vi "Config Dialog.vi"(10 "Container State":T2 caption="container state", 11 "state in":T3={"Draw Options"={"Text Color"=16777238, "Wing Color"=16751616, "Dial Outline Color"=13816530, "Sky Color"=3381759, "Ground Color"=8213043, "Horizon Line Color"=16777225, "Outline Color"=0, "Dial Background Color"=5987163, "Draw Wings"=TRUE, "Draw Text"=TRUE, "Font Name"="Helvetica", "Angle units"=enum."Radians"}} caption="State") -> (0 "state changed?":bool, 1 "data changed?":bool, 3 "state out":T3={"Draw Options"={"Text Color"=16777238, "Wing Color"=16751616, "Dial Outline Color"=13816530, "Sky Color"=3381759, "Ground Color"=8213043, "Horizon Line Color"=16777225, "Outline Color"=0, "Dial Background Color"=5987163, "Draw Wings"=TRUE, "Draw Text"=TRUE, "Font Name"="Helvetica", "Angle units"=enum."Radians"}} caption="State")   [LabVIEW 2017, in "Attitude Indicator.xctl"]
uses:
  <vilib>/robotics/Controls/Attitude Indicator/Attitude Indicator.xctl
  <vilib>/robotics/Controls/Utilities/Color Box_No Transparent.ctl
  <vilib>/robotics/Controls/Utilities/Color Box.ctl
  <vilib>/robotics/Controls/Attitude Indicator/_Attitude Indicator Support Files/Attitude Indicator State.ctl
  <vilib>/robotics/Controls/Attitude Indicator/Attitude Picture/Draw Options.ctl
  <vilib>/robotics/Controls/Utilities/Angle Units.ctl
  <vilib>/_xctls/Container State.ctl
  <vilib>/robotics/Controls/Attitude Indicator/Attitude Picture/Attitude.ctl
  <vilib>/robotics/Controls/Attitude Indicator/Attitude Picture/NI_Robotics_Attitude Picture.lvlib
  <vilib>/_xctls/XControlSupport.lvlib
  <vilib>/robotics/Controls/Utilities/NI_Robotics_Control Utilities.lvlib
panel:
  in  "help":bool
  in  "cancel":bool
  in  "ok":bool
  in  "Angle Units":enum16{"Radians", "Degrees"}(ring)=enum."Degrees"
  in  "text":T1=16777238 caption="Text"
  out "2D Picture":picture
  in  "dial outline color":T1=13816530 caption="Dial Outline"
  in  "draw text":bool=TRUE caption="Draw Text"
  in  "draw wings":bool=TRUE caption="Draw Wings"
  in  "dial bkgnd color":T6=5987163 caption="Dial Background"
  in  "outline color":T6 caption="Outline"
  in  "horizon line color":T1=16777225 caption="Horizon Line"
  in  "ground color":T1=8213043 caption="Ground"
  in  "sky color":T1=3381759 caption="Sky"
  in  "wing color":T1=16751616 caption="Wings"
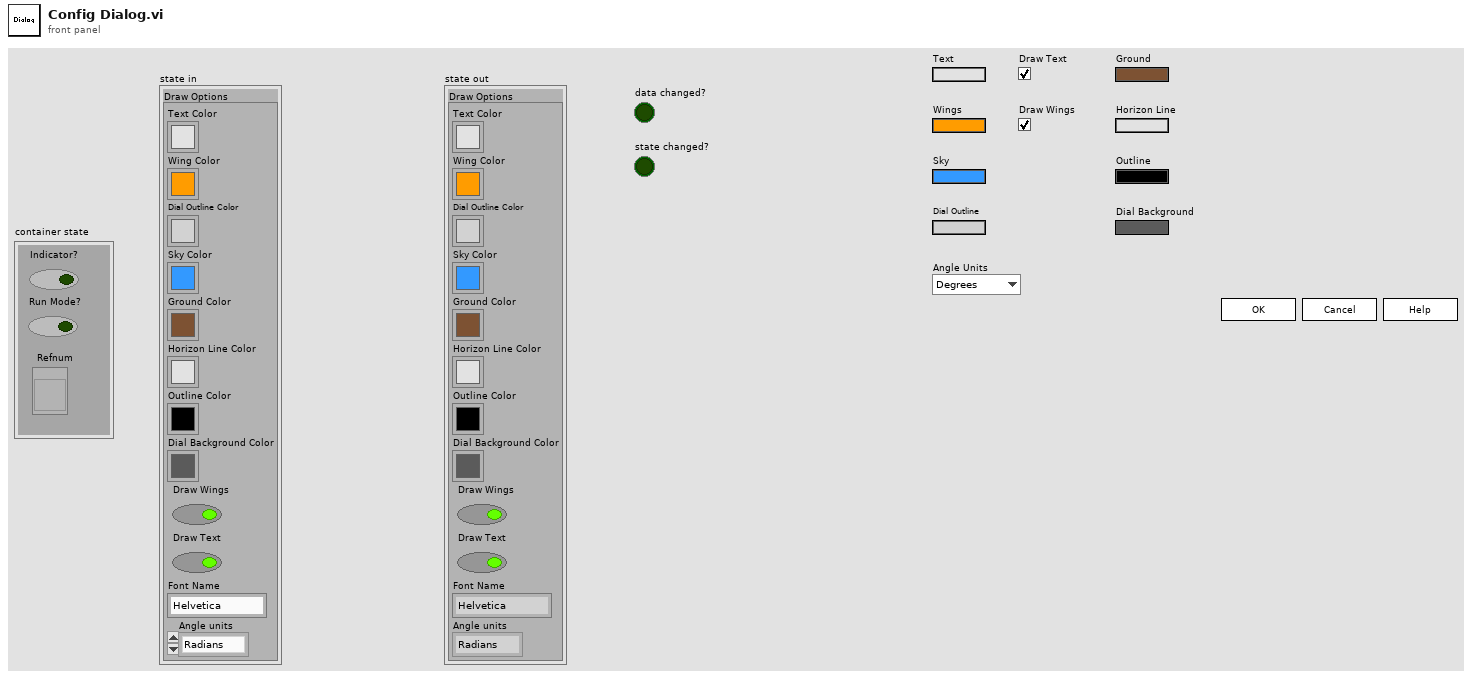
[diagram p1: front panel]
types:
  T1 = typedef "NI_Robotics_Control Utilities.lvlib/Color Box_No Transparent.ctl" = u32
  T2 = typedef "XControlSupport.lvlib/Container State.ctl" = cluster{"Indicator?":bool, "Run Mode?":bool, " Refnum":refnum<vi>}
  T3 = typedef "Attitude Indicator.xctl/Attitude Indicator State.ctl" = cluster{"Draw Options":T4}
  T4 = typedef "NI_Robotics_Attitude Picture.lvlib/Draw Options.ctl" = cluster{"Text Color":u32, "Wing Color":u32, "Dial Outline Color":u32, "Sky Color":u32, "Ground Color":u32, "Horizon Line Color":u32, "Outline Color":u32, "Dial Background Color":u32, "Draw Wings":bool, "Draw Text":bool, "Font Name":string, "Angle units":T5}
  T5 = typedef "NI_Robotics_Control Utilities.lvlib/Angle Units.ctl" = enum16{"Radians", "Degrees"}
  T6 = typedef "NI_Robotics_Control Utilities.lvlib/Color Box.ctl" = u32
  T7 = typedef "NI_Robotics_Attitude Picture.lvlib/Attitude.ctl" = cluster{"roll":dbl, "pitch":dbl}
  T8 = typedef "LVBoundsTypeDef.ctl" = cluster{"Width":u32, "Height":u32}
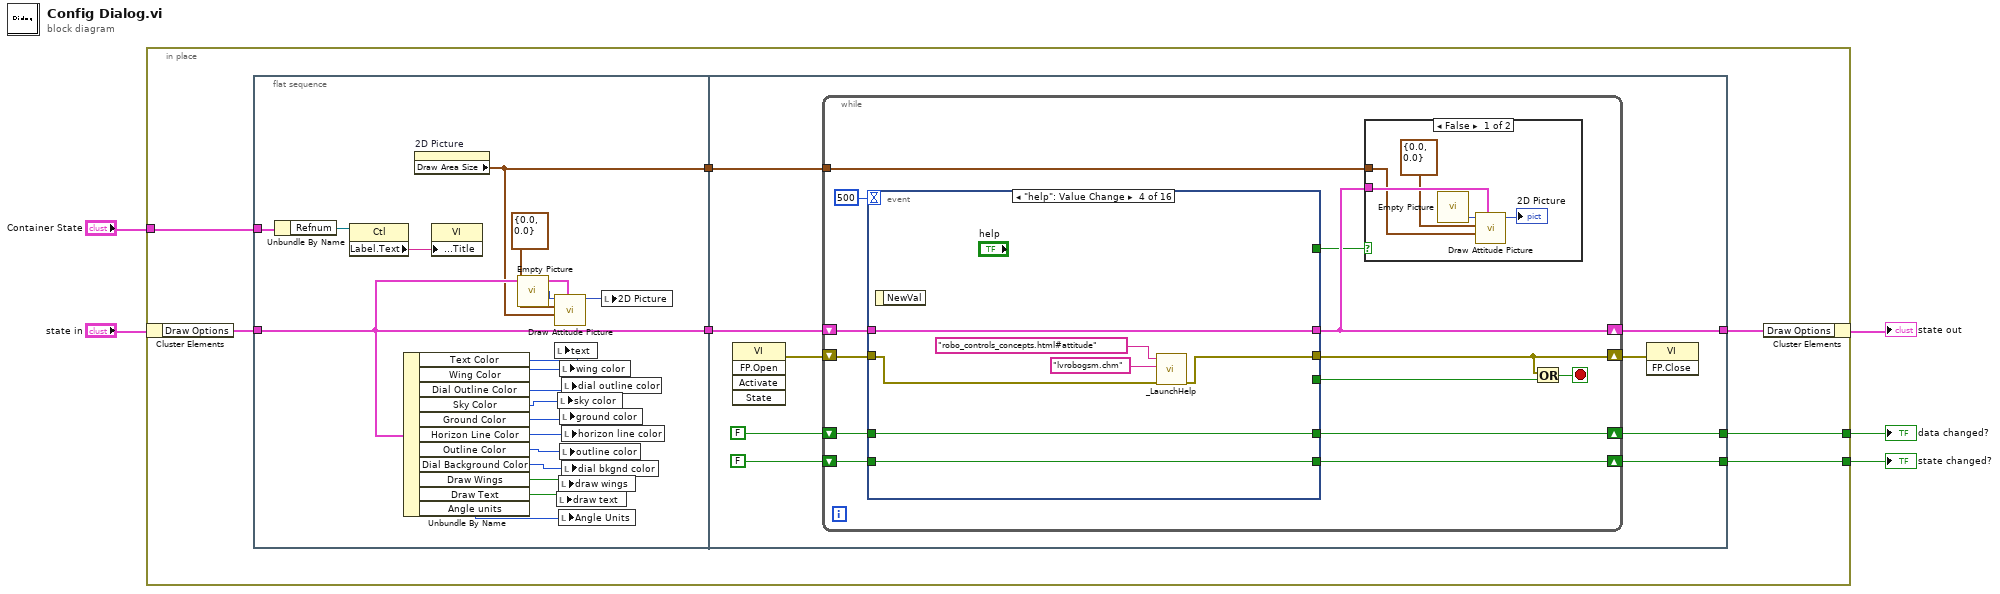
[diagram p0: block diagram]
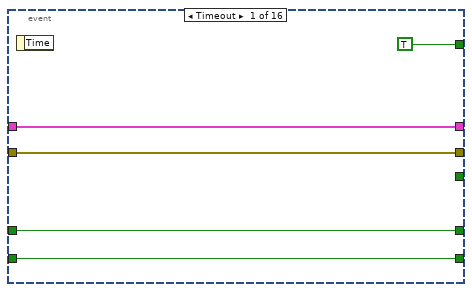
[diagram p3: hidden frame]
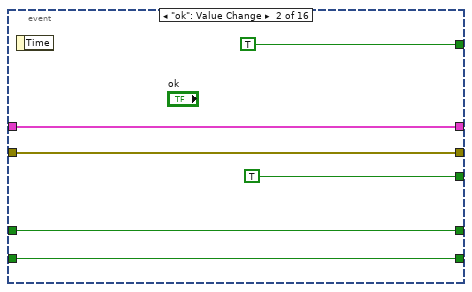
[diagram p4: hidden frame]
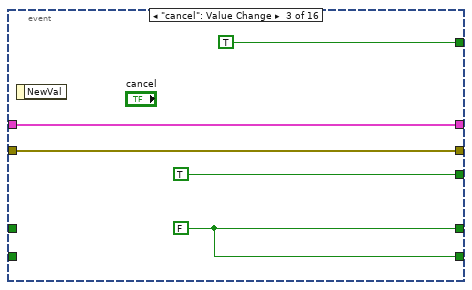
[diagram p5: hidden frame]
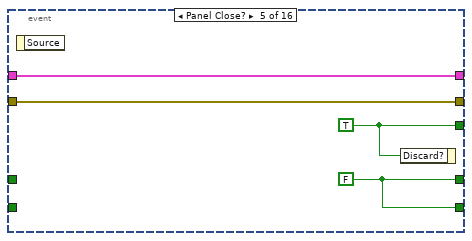
[diagram p6: hidden frame]
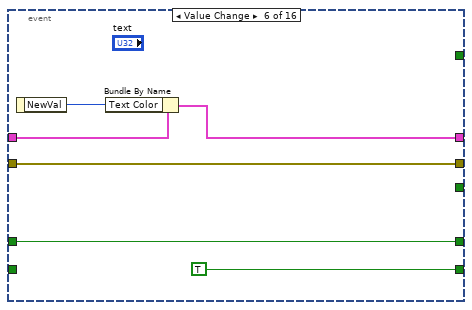
[diagram p7: hidden frame]
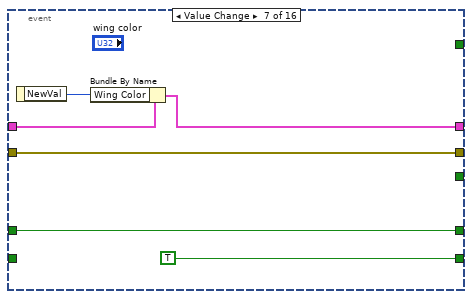
[diagram p8: hidden frame]
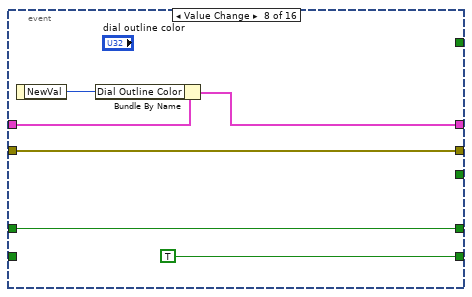
[diagram p9: hidden frame]
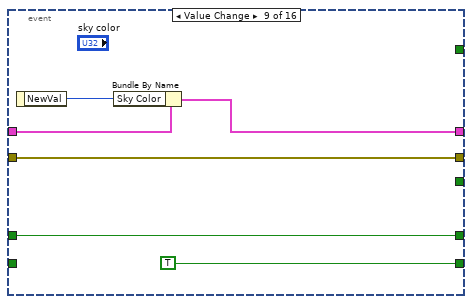
[diagram p10: hidden frame]
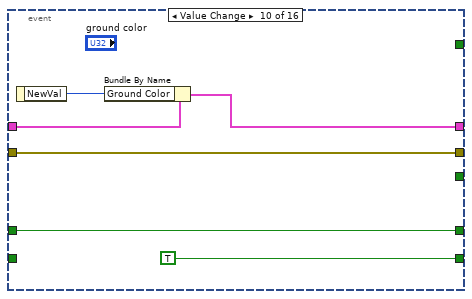
[diagram p11: hidden frame]
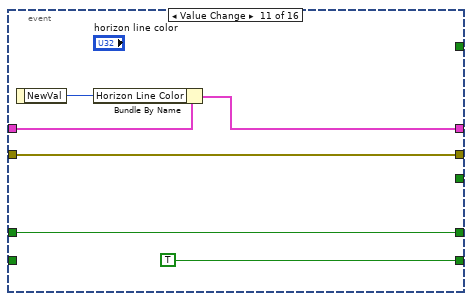
[diagram p12: hidden frame]
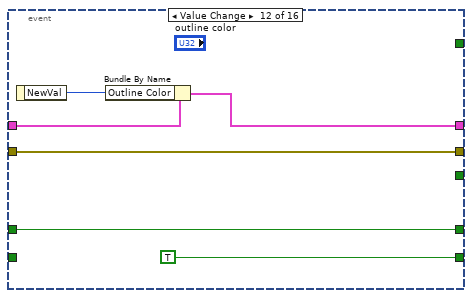
[diagram p13: hidden frame]
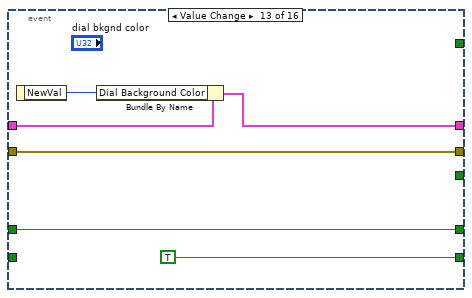
[diagram p14: hidden frame]
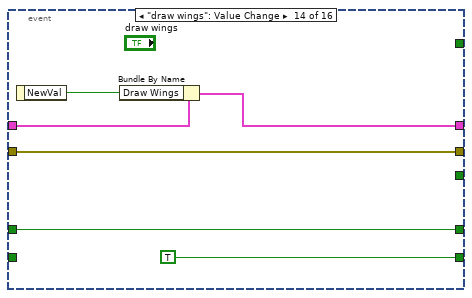
[diagram p15: hidden frame]
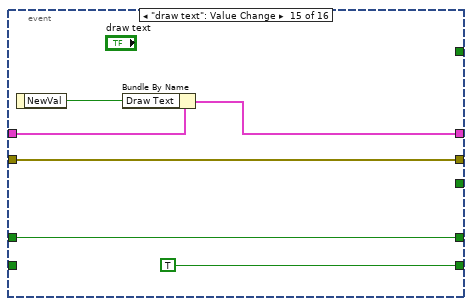
[diagram p16: hidden frame]
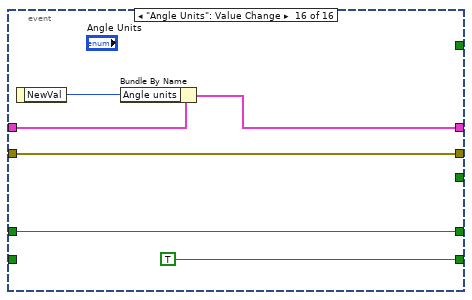
[diagram p17: hidden frame]
diagram:
  n1 = in-place {
    in-place-border: [w10] -> w5
    in-place-border: [w9] -> w4
    in-place-border: "Container State" -> [w6]
    n2 = in-place-cluster #1("state in") -> ("Draw Options"=w8:T4)
    n3 = flat-sequence {
      tunnel: w8 -> [w20]
      tunnel: [w20] -> w12
      tunnel: [w19] -> w11
      tunnel: w6 -> [w17]
      tunnel: [w39] -> w7
      tunnel: w12 -> [w40]
      tunnel: [w34] -> w10
      tunnel: [w33] -> w9
      tunnel: w11 -> [w32]
      frame #0 {
        n4 = Unbundle By Name(w17) -> ("Refnum"=w16:refnum<vi>)
        n5 = property class="Ctl"(reference=w16) -> ("Label.Text"=w15:string)  [unwired: 1 in, 2 out]
        n6 = Unbundle By Name(w20) -> ("Text Color"=w31:u32, "Wing Color"=w30:u32, "Dial Outline Color"=w29:u32, "Sky Color"=w28:u32, "Ground Color"=w27:u32, "Horizon Line Color"=w26:u32, "Outline Color"=w25:u32, "Dial Background Color"=w24:u32, "Draw Wings"=w23:bool, "Draw Text"=w22:bool, "Angle units"=w14:T5)
        n7 = property on="2D Picture" class="Pict"() -> ("Draw Area Size"=w19:T8)  [unwired: 2 in, 2 out]
        n8 = property class="VI"("Front Panel.Title"=w15) -> ()  [unwired: 2 in, 2 out]
        n9 = call "Empty Picture"() -> ("empty picture"=w18:picture)
        n10 = call <vilib>:"Draw Attitude Picture.vi"("draw options"=w20, "DrawAreaSize"=w19, "attitude"=T7 {"roll"=0.0, "pitch"=0.0}, "picture in"=w18) -> ("picture out"=w21:picture)  [unwired: 6 in, 1 out]
        n11 = local write "text"(w31) -> ()
        n12 = local write "draw text"(w22) -> ()
        n13 = local write "sky color"(w28) -> ()
        n14 = local write "draw wings"(w23) -> ()
        n15 = local write "Angle Units"(w14) -> ()
        n16 = local write "wing color"(w30) -> ()
        n17 = local write "ground color"(w27) -> ()
        n18 = local write "outline color"(w25) -> ()
        n19 = local write "dial outline color"(w29) -> ()
        n20 = local write "horizon line color"(w26) -> ()
        n21 = local write "dial bkgnd color"(w24) -> ()
        n22 = local write "2D Picture"(w21) -> ()
      }
      frame #1 {
        n23 = invoke class="VI" method="FP.Open"() -> (error out=w38:errorcluster)  [unwired: 5 in, 4 out]
        n24 = while {
          shift-right: [w42] -> w39
          shift-left: w40 -> [w53]
          shift-right: [w48] -> w35
          shift-left: w38 -> [w51]
          shift-right: [w44] -> w34
          shift-left: FALSE -> [w50]
          shift-right: [w45] -> w33
          shift-left: FALSE -> [w49]
          tunnel: w32 -> [w43]
          stop <- w46 stop-if-true
          n25 = event shown="[3] \"help\": Value Change" {
            selector: _ -> [_ _ _ _ _ _ _ _ _ _ _ _ _ _ _ _]
            dyn-events: _ -> [_ _ _ _ _ _ _ _ _ _ _ _ _ _ _ _]
            timeout: 500 -> [_ _ _ _ _ _ _ _ _ _ _ _ _ _ _ _]
            tunnel: w53 -> [w63 w69 w74 w81 w85 w90 w94 w100 w106 w112 w118 w124 w130 w136 w142 w148]
            tunnel: w51 -> [w62 w68 w73 w76 w84 w88 w97 w103 w109 w115 w121 w127 w133 w139 w145 w151]
            tunnel: w50 -> [w61 w66 _ w79 _ w87 w96 w102 w108 w114 w120 w126 w132 w138 w144 w150]
            tunnel: w49 -> [w60 w67 _ w80 _ _ _ _ _ _ _ _ _ _ _ _]
            tunnel: [w63 w69 w74 w81 w85 w89 w93 w99 w105 w111 w117 w123 w129 w135 w141 w147] -> w42
            tunnel: [w62 w68 w73 w75 w84 w88 w97 w103 w109 w115 w121 w127 w133 w139 w145 w151] -> w48
            tunnel: [_ TRUE TRUE _ w83 _ _ _ _ _ _ _ _ _ _ _] -> w47
            tunnel: [w60 w67 w71 w80 w82 TRUE TRUE TRUE TRUE TRUE TRUE TRUE TRUE TRUE TRUE TRUE] -> w45
            tunnel: [w61 w66 w71 w79 w82 w87 w96 w102 w108 w114 w120 w126 w132 w138 w144 w150] -> w44
            tunnel: [TRUE TRUE TRUE _ _ _ _ _ _ _ _ _ _ _ _ _] -> w41
            event Timeout {
              n26 = event-data() -> ()  [unwired: 1 in, 1 out]
            }
            event "ok": Value Change {
              n27 = event-data() -> ()  [unwired: 1 in, 1 out]
            }
            event "cancel": Value Change {
              w71 = FALSE
              n28 = event-data() -> ()  [unwired: 1 in, 1 out]
            }
            event "help": Value Change {
              n29 = event-data() -> ()  [unwired: 1 in, 1 out]
              n30 = call <helpdir>:"_LaunchHelp.vi"("error in (no error)"=w76, "CHM or HLP filename (lvdialog.chm)"="lvrobogsm.chm", "HTML filename"="robo_controls_concepts.html#attitude") -> ("error out"=w75:errorcluster)  [unwired: 4 out]
            }
            event Panel Close? {
              w82 = FALSE
              w83 = TRUE
              n31 = event-data() -> ()  [unwired: 1 in, 1 out]
              n32 = event-data("Discard?"=w83) -> ()  [unwired: 1 in, 1 out]
            }
            event Value Change {
              n33 = event-data() -> ("NewVal"=w91:T1)  [unwired: 1 in]
              n34 = Bundle By Name(cluster=w90, "Text Color"=w91) -> (w89:T4)
            }
            event Value Change {
              n35 = event-data() -> ("NewVal"=w95:T1)  [unwired: 1 in]
              n36 = Bundle By Name(cluster=w94, "Wing Color"=w95) -> (w93:T4)
            }
            event Value Change {
              n37 = event-data() -> ("NewVal"=w101:T1)  [unwired: 1 in]
              n38 = Bundle By Name(cluster=w100, "Dial Outline Color"=w101) -> (w99:T4)
            }
            event Value Change {
              n39 = event-data() -> ("NewVal"=w107:T1)  [unwired: 1 in]
              n40 = Bundle By Name(cluster=w106, "Sky Color"=w107) -> (w105:T4)
            }
            event Value Change {
              n41 = event-data() -> ("NewVal"=w113:T1)  [unwired: 1 in]
              n42 = Bundle By Name(cluster=w112, "Ground Color"=w113) -> (w111:T4)
            }
            event Value Change {
              n43 = event-data() -> ("NewVal"=w119:T1)  [unwired: 1 in]
              n44 = Bundle By Name(cluster=w118, "Horizon Line Color"=w119) -> (w117:T4)
            }
            event Value Change {
              n45 = event-data() -> ("NewVal"=w125:T6)  [unwired: 1 in]
              n46 = Bundle By Name(cluster=w124, "Outline Color"=w125) -> (w123:T4)
            }
            event Value Change {
              n47 = event-data() -> ("NewVal"=w131:T6)  [unwired: 1 in]
              n48 = Bundle By Name(cluster=w130, "Dial Background Color"=w131) -> (w129:T4)
            }
            event "draw wings": Value Change {
              n49 = event-data() -> ("NewVal"=w137:bool)  [unwired: 1 in]
              n50 = Bundle By Name(cluster=w136, "Draw Wings"=w137) -> (w135:T4)
            }
            event "draw text": Value Change {
              n51 = event-data() -> ("NewVal"=w143:bool)  [unwired: 1 in]
              n52 = Bundle By Name(cluster=w142, "Draw Text"=w143) -> (w141:T4)
            }
            event "Angle Units": Value Change {
              n53 = event-data() -> ("NewVal"=w149:enum16{"Radians", "Degrees"})  [unwired: 1 in]
              n54 = Bundle By Name(cluster=w148, "Angle units"=w149) -> (w147:T4)
            }
          }
          n55 = case shown="False" w41 {
            tunnel: w43 -> [w56 _]
            tunnel: w42 -> [w57 _]
            frame False {
              n56 = call "Empty Picture"() -> ("empty picture"=w55:picture)
              n57 = call <vilib>:"Draw Attitude Picture.vi"("draw options"=w57, "DrawAreaSize"=w56, "attitude"=T7 {"roll"=0.0, "pitch"=0.0}, "picture in"=w55) -> ("picture out"=→"2D Picture":picture)  [unwired: 6 in, 1 out]
            }
            frame True {
            }
          }
          n58 = Or(x=w48, y=w47) -> (x .or. y?=w46:bool)
        }
        n59 = invoke class="VI" method="FP.Close"(error in=w35) -> ()  [unwired: 2 in, 3 out]
      }
    }
    n60 = in-place-cluster #1("Draw Options"=w7) -> (→"state out":T3)
  }
  "data changed?" <- w5
  "state changed?" <- w4
